vi "SMBUS Block Process Call.vi"(0 "DevHandle":i32, 1 "pWriteData":string, 2 "pReadData":string, 3 "WithPEC":u8, 5 "IICIndex":i32, 7 "SlaveAddr":i16, 9 "CommandCode":u8, 12 "WriteCount":i32, 13 "pReadCount":i32) -> (4 "pWriteData out":string, 6 "pReadData out":string, 8 "pReadCount out":i32, 10 "function return":i32)   [LabVIEW 2010, in "usb2iic.lvlib"]
doc: "int WINAPI SMBUS_BlockProcessCall(int DevHandle,int IICIndex,short SlaveAddr,unsigned char CommandCode, unsigned char *pWriteData,int WriteCount, unsigned char *pReadData,int *pReadCount,unsigned char WithPEC);"
uses:
  usb2iic.lvlib
  USB2XXX.dll
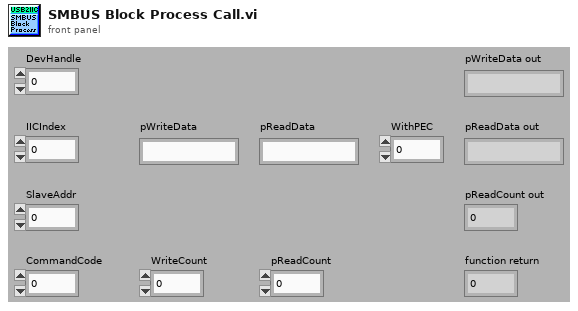
[diagram p1: front panel]
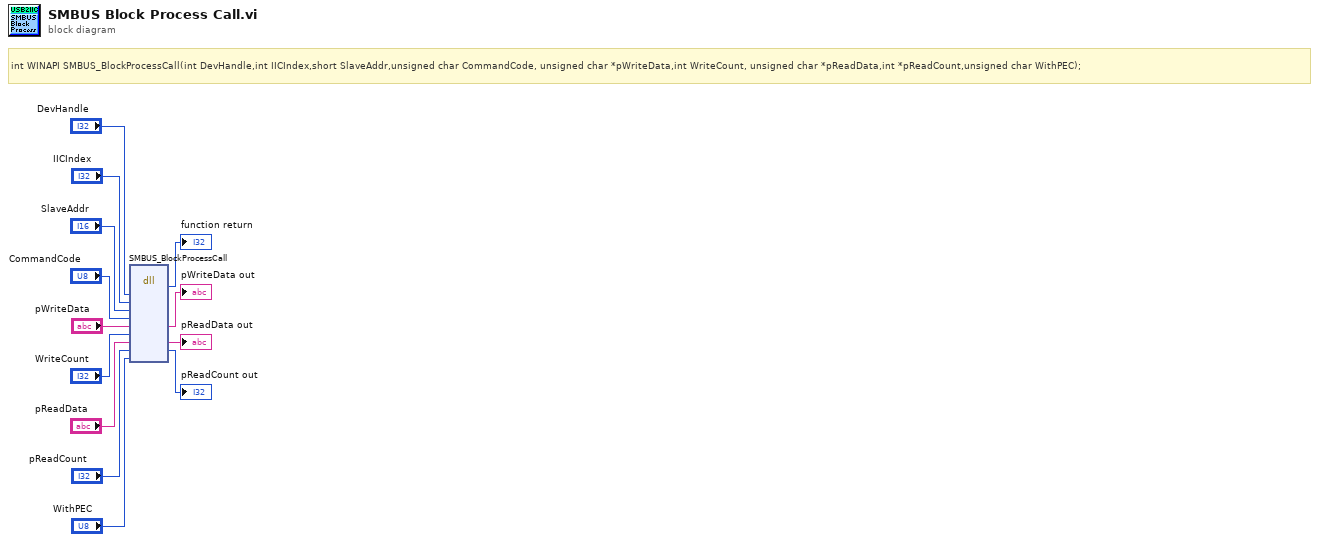
[diagram p0: block diagram]
diagram:
  # "int WINAPI SMBUS_BlockProcessCall(int DevHandle,int IICIndex,short SlaveAddr,unsigned char CommandCode, unsigned char *pWriteData,int WriteCount, unsigned char *pReadData,int *pReadCount,unsigned char WithPEC);"
  n1 = dll-call lib="G:/OtherWork/USB2XXX_Example/trunk/Labview/PublicFiles/USB2XXX.*" fn="SMBUS_BlockProcessCall"("DevHandle"="DevHandle", "IICIndex"="IICIndex", "SlaveAddr"="SlaveAddr", "CommandCode"="CommandCode", "pWriteData"="pWriteData", "WriteCount"="WriteCount", "pReadData"="pReadData", "pReadCount"="pReadCount", "WithPEC"="WithPEC") -> (→"function return":i32, "pWriteData"=→"pWriteData out":string, "pReadData"=→"pReadData out":string, "pReadCount"=→"pReadCount out":i32)  [unwired: 9 in, 2 out]
